vi "Filter Empty Lines.vi"(0 "Functions in":T1[](array[typedef]), 11 "error in (no error)":errorcluster) -> (4 "Functions":T1[](array[typedef]), 15 "error out":errorcluster)   [LabVIEW 2019]
uses:
  Line Details.ctl
  <vilib>/Utility/error.llb/whitespace.ctl
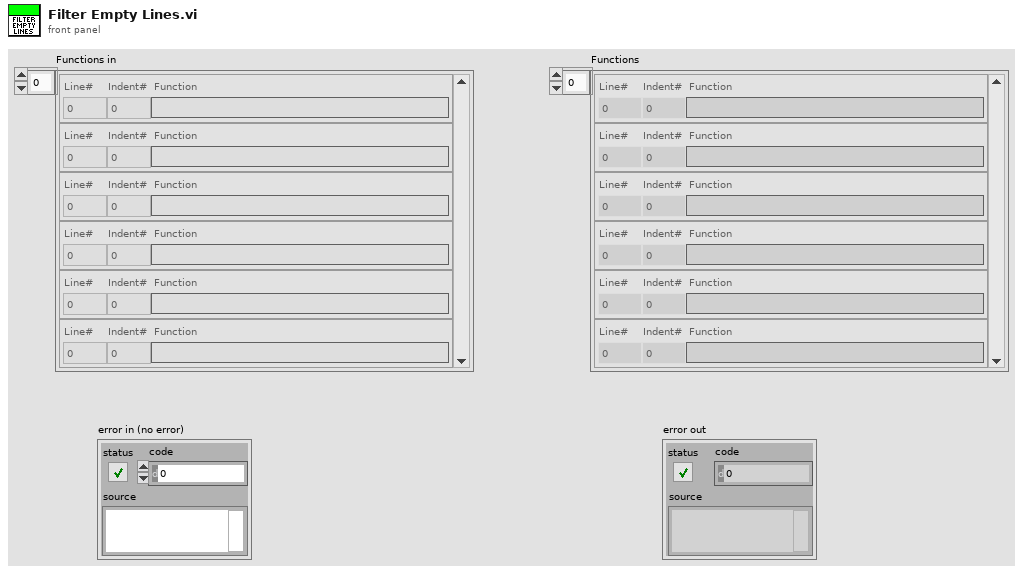
[diagram p1: front panel]
types:
  T1 = typedef "Line Details.ctl" = cluster{"Line#":i64, "Indent#":i64, "Function":string}
  T2 = typedef "whitespace.ctl" = u16
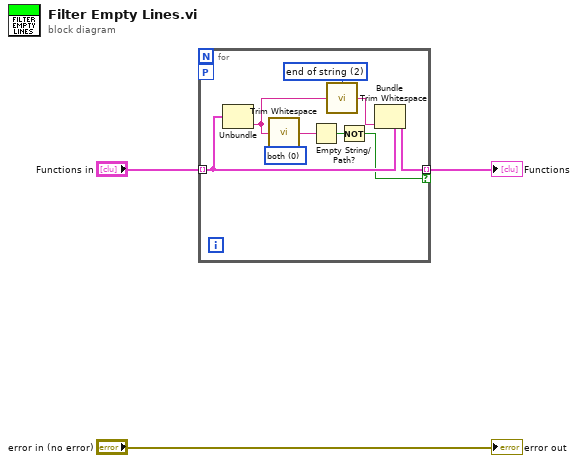
[diagram p0: block diagram]
diagram:
  n1 = for {
    tunnel: "Functions in" -> [w10] mode=indexing
    tunnel: [w8] -> w1 mode=indexing if=w7
    workers-P: _ -> [_]
    w6 = T2 2 items=["both", "start of string", "end of string"] ("location (both)")
    w11 = T2 0 items=["both", "start of string", "end of string"] ("location (both)")
    n2 = Unbundle(w10) -> ("Function"=w4:string)  [unwired: 2 out]
    n3 = call <vilib>:"Trim Whitespace.vi"("string"=w4, "location (both)"=w11) -> ("trimmed string"=w9:string)
    n4 = Empty String/Path?(string/path=w9) -> (empty?=w12:bool)
    n5 = call <vilib>:"Trim Whitespace.vi"("string"=w4, "location (both)"=w6) -> ("trimmed string"=w5:string)
    n6 = Not(x=w12) -> (.not. x?=w7:bool)
    n7 = Bundle(cluster=w10, "Function"=w5) -> (w8:T1)  [unwired: 2 in]
  }
  "Functions" <- w1
  "error out" <- "error in (no error)"
